vi "WLAN - niVST - RFSG - GenAndWriteWfm.vi"(8 "Address String":string="00:90:4C:C5:12:38", 9 "WaveformNamePostfix":string, 10 "Rx Measurements Settings":T1={"Channel Bandwidth (Hz)"=4.0, "Idle Interval (s)"=40000000.0, "MCS Index"=0, "80211n PLCP Frame Format"=0, "Payload Data Length (bytes)"=0, "OFDM Data Rate (Mbps)"=1024, "DSSS Data Rate (Mbps)"=0, "#N_SS"=0, "NIStandard"=enum."80211A/G/J/P(OFDM)"} {"DSSS Data Rate (Mbps)" items=["1", "2", "5.5 CCK", "5.5 PBCC", "11 CCK", "11 PBCC", "22", "33"]; "OFDM Data Rate (Mbps)" items=["6", "9", "12", "18", "24", "36", "48", "54"]; "80211n PLCP Frame Format" items=["Mixed Format", "Greenfield Format"]}, 11 "instrument handle":refnum<k15>="pxi1slot2") -> (0 "error out":errorcluster, 3 "RFSG out":refnum<k15>)   [LabVIEW 2012]
uses:
  TV/RW/Includes/WLAN - TV - OPPO - RW - INC - TV_Rx_Measurements.ctl
  TV/RW/Includes/WLAN - NIStandardDefine.ctl
  <instrlib>/niRFSG/niRFSG.llb/niRFSG Ref Clock Sources.ctl
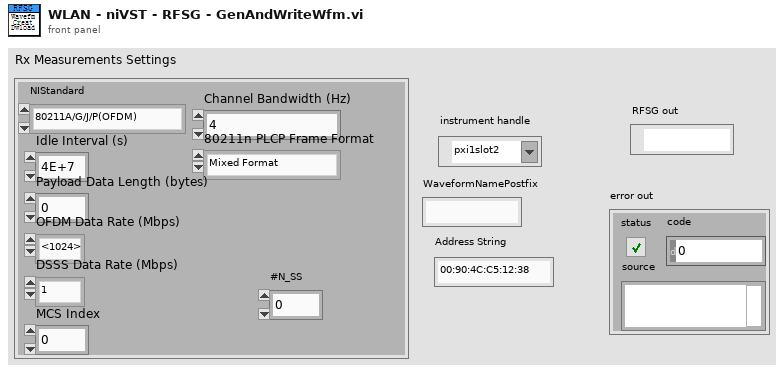
[diagram p1: front panel]
types:
  T1 = typedef "WLAN - TV - OPPO - RW - INC - TV_Rx_Measurements.ctl" = cluster{"Channel Bandwidth (Hz)":dbl, "Idle Interval (s)":dbl, "MCS Index":i32, "80211n PLCP Frame Format":i32, "Payload Data Length (bytes)":i32, "OFDM Data Rate (Mbps)":i32, "DSSS Data Rate (Mbps)":i32, "#N_SS":i32, "NIStandard":T2}
  T2 = typedef "WLAN - NIStandardDefine.ctl" = enum32{"80211A/G/J/P(OFDM)", "80211B/G(DSSS)", "80211GDSSSOFDM", "80211NMIMOOFDM", "80211ACMIMOOFDM"}
  T3 = typedef "niRFSG Ref Clock Sources.ctl" = string
  T4 = typedef "WLAN - TV - RW - INC - Rx_PER_Wfm_Settings.ctl" = cluster{"Standard":i32, "Channel Bandwidth (Hz)":dbl, "Idle Interval (s)":dbl, "MCS Index":i32, "80211n PLCP Frame Format":i32, "Payload Data Length (bytes)":i32, "OFDM Data Rate (Mbps)":i32, "DSSS Data Rate (Mbps)":i32, "Wfm_Index":i32, "#N_SS":i32}
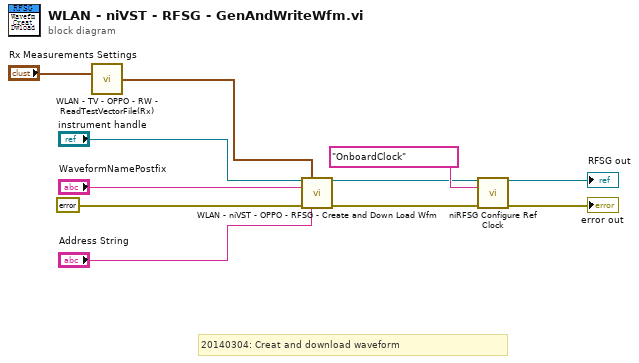
[diagram p0: block diagram]
diagram:
  # "20140304: Creat and download waveform"
  n1 = call "WLAN - TV - OPPO - RW - ReadTestVectorFile(Rx).vi"("Rx Measurements Settings"="Rx Measurements Settings") -> ("Waveform Generation Settings"=w10:T4)  [unwired: 14 in]
  n2 = call "WLAN - niVST - OPPO - RFSG - Create and Down Load Wfm.vi"("instrument handle"="instrument handle", "Waveform Generation Settings"=w10, "WaveformNamePostfix"="WaveformNamePostfix", "error in"=errorcluster {"status"=FALSE, "code"=0, "source"=""}, "Address String"="Address String") -> ("instrument handle"=w6:refnum<k15>, "error out"=w5:errorcluster)  [unwired: 8 in, 1 out]
  n3 = call <instrlib>:"niRFSG Configure Ref Clock.vi"("instrument handle"=w6, "ref clock source"=T3 "OnboardClock", "error in"=w5) -> ("instrument handle out"=→"RFSG out":refnum<k15>, "error out"=→"error out":errorcluster)  [unwired: 11 out]
